vi "Flancos.vi"() -> ()   [LabVIEW 2017]
panel:
  out "Falling 4":dbl
  out "Rise 4":dbl
  out "Falling 3":dbl
  out "Rise 3":dbl
  out "Falling 2":dbl
  out "Rise 2":dbl
  out "Falling":dbl
  out "Rise":dbl
  in  "stop":bool
  in  "Alarma 4":bool
  in  "Alarma 3":bool
  in  "Alarma 2":bool
  in  "Alarma":bool
  out "Conteo 4":bool
  out "Conteo 3":bool
  out "Conteo 2":bool
  in  "stop 2":bool
  out "Waveform Chart":dbl(graph)
  in  "Seleccion":bool
  out "Conteo":bool
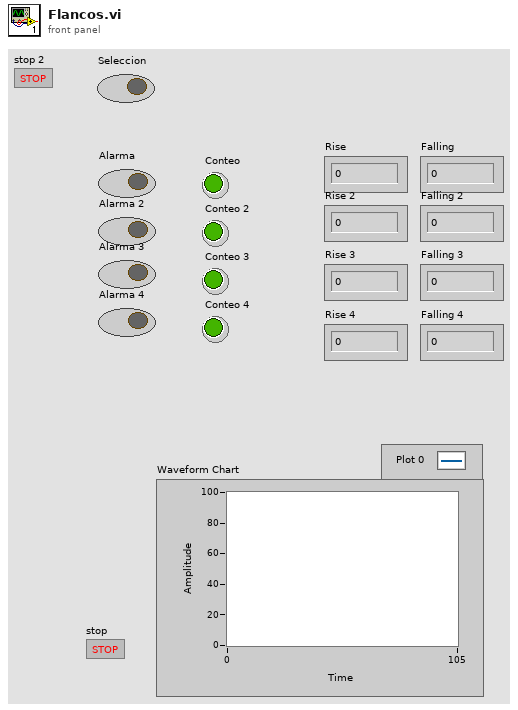
[diagram p1: front panel]
types:
  T1 = cluster{"Cont":i32, "Cont2":i32, "Cont3":i32, "Cont4":i32, "Bajada":i32, "Bajada 2":i32, "Bajada 3":i32, "Bajada 4":i32}
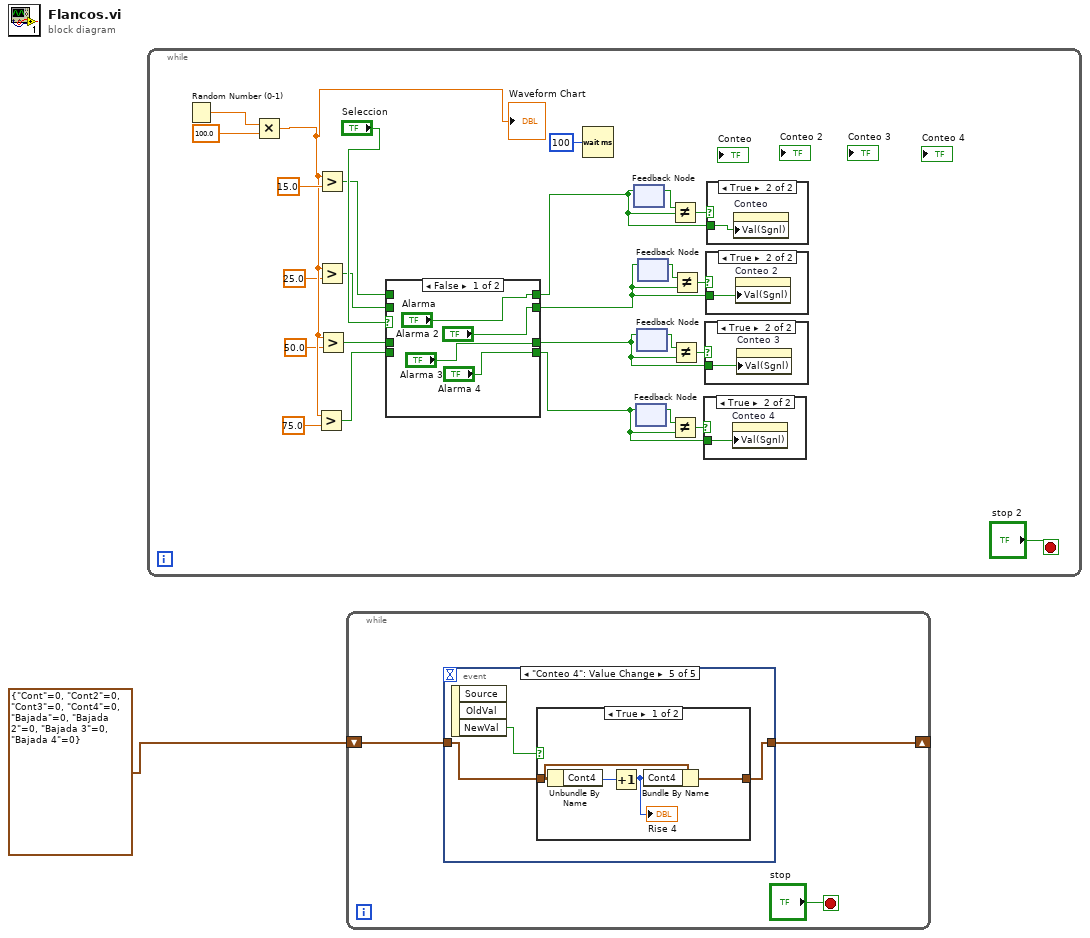
[diagram p0: block diagram]
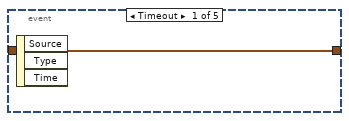
[diagram p2: hidden frame]
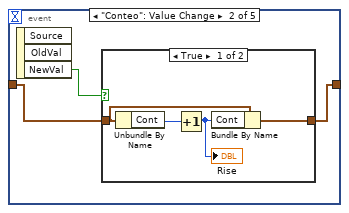
[diagram p3: hidden frame]
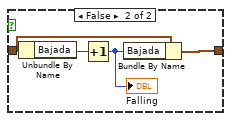
[diagram p4: hidden frame]
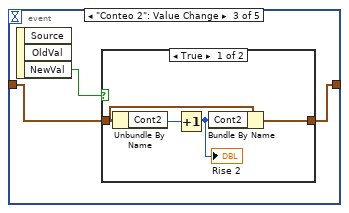
[diagram p5: hidden frame]
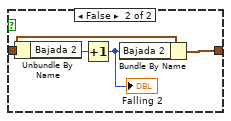
[diagram p6: hidden frame]
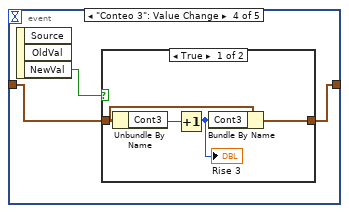
[diagram p7: hidden frame]
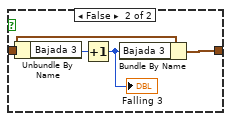
[diagram p8: hidden frame]
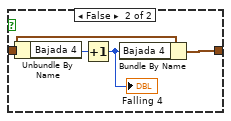
[diagram p9: hidden frame]
diagram:
  n1 = while {
    stop <- "stop 2" stop-if-true
    n2 = Random Number (0-1)() -> (number: 0 to 1=w27:dbl)
    n3 = Multiply(x=w27, y=100.0) -> (x*y=w20:dbl)
    "Waveform Chart" <- w20
    n4 = Greater?(x=w20, y=75.0) -> (0:w12:bool)
    n5 = Greater?(x=w20, y=15.0) -> (0:w15:bool)
    n6 = Greater?(x=w20, y=25.0) -> (0:w14:bool)
    n7 = Greater?(x=w20, y=50.0) -> (0:w13:bool)
    n8 = case shown="False" "Seleccion" {
      tunnel: w15 -> [_ w38]
      tunnel: w14 -> [_ w37]
      tunnel: w13 -> [_ w36]
      tunnel: w12 -> [_ w35]
      tunnel: ["Alarma" w38] -> w11
      tunnel: ["Alarma 2" w37] -> w8
      tunnel: ["Alarma 3" w36] -> w5
      tunnel: ["Alarma 4" w35] -> w2
      frame False {
      }
      frame True {
      }
    }
    n9 = Wait (ms)(milliseconds to wait=u32 100) -> ()  [unwired: 1 out]
    n10 = feedback-in #1(w11) -> ()
    n11 = feedback #1() -> (w22:bool)  [unwired: 1 in]
    n12 = feedback #2() -> (w4:bool)  [unwired: 1 in]
    n13 = feedback-in #2(w2) -> ()
    n14 = feedback #3() -> (w7:bool)  [unwired: 1 in]
    n15 = feedback-in #3(w5) -> ()
    n16 = feedback #4() -> (w10:bool)  [unwired: 1 in]
    n17 = feedback-in #4(w8) -> ()
    n18 = Not Equal?(x=w22, y=w11) -> (x != y?=w21:bool)
    n19 = Not Equal?(x=w4, y=w2) -> (x != y?=w3:bool)
    n20 = Not Equal?(x=w7, y=w5) -> (x != y?=w6:bool)
    n21 = Not Equal?(x=w10, y=w8) -> (x != y?=w9:bool)
    n22 = case shown="True" w3 {
      tunnel: w2 -> [_ w28]
      frame False {
      }
      frame True {
        n23 = property on="Conteo 4" class="Bool (strict)"("Val(Sgnl)"=w28) -> ()  [unwired: 2 in, 2 out]
      }
    }
    n24 = case shown="True" w6 {
      tunnel: w5 -> [_ w29]
      frame False {
      }
      frame True {
        n25 = property on="Conteo 3" class="Bool (strict)"("Val(Sgnl)"=w29) -> ()  [unwired: 2 in, 2 out]
      }
    }
    n26 = case shown="True" w9 {
      tunnel: w8 -> [_ w30]
      frame False {
      }
      frame True {
        n27 = property on="Conteo 2" class="Bool (strict)"("Val(Sgnl)"=w30) -> ()  [unwired: 2 in, 2 out]
      }
    }
    n28 = case shown="True" w21 {
      tunnel: w11 -> [_ w39]
      frame False {
      }
      frame True {
        n29 = property on="Conteo" class="Bool (strict)"("Val(Sgnl)"=w39) -> ()  [unwired: 2 in, 2 out]
      }
    }
  }
  n30 = while {
    shift-right: [w40] -> _
    shift-left: T1 {"Cont"=0, "Cont2"=0, "Cont3"=0, "Cont4"=0, "Bajada"=0, "Bajada 2"=0, "Bajada 3"=0, "Bajada 4"=0} -> [w42]
    stop <- "stop" stop-if-true
    n31 = event shown="[4] \"Conteo 4\": Value Change" {
      selector: _ -> [_ _ _ _ _]
      dyn-events: _ -> [_ _ _ _ _]
      timeout: _ -> [_ _ _ _ _]
      tunnel: w42 -> [w43 w46 w57 w68 w79]
      tunnel: [w43 w45 w56 w67 w78] -> w40
      event Timeout {
        n32 = event-data() -> ()  [unwired: 1 in, 3 out]
      }
      event "Conteo": Value Change {
        n33 = event-data() -> ("NewVal"=w44:bool)  [unwired: 1 in, 2 out]
        n34 = case shown="True" w44 {
          tunnel: w46 -> [w49 w53]
          tunnel: [w48 w52] -> w45
          frame True {
            n35 = Unbundle By Name(w49) -> ("Cont"=w50:i32)
            n36 = Increment(x=w50) -> (x+1=w47:i32)
            "Rise" <- w47
            n37 = Bundle By Name(cluster=w49, "Cont"=w47) -> (w48:T1)
          }
          frame False {
            n38 = Unbundle By Name(w53) -> ("Bajada"=w54:i32)
            n39 = Increment(x=w54) -> (x+1=w51:i32)
            "Falling" <- w51
            n40 = Bundle By Name(cluster=w53, "Bajada"=w51) -> (w52:T1)
          }
        }
      }
      event "Conteo 2": Value Change {
        n41 = event-data() -> ("NewVal"=w55:bool)  [unwired: 1 in, 2 out]
        n42 = case shown="True" w55 {
          tunnel: w57 -> [w60 w64]
          tunnel: [w59 w63] -> w56
          frame True {
            n43 = Unbundle By Name(w60) -> ("Cont2"=w61:i32)
            n44 = Increment(x=w61) -> (x+1=w58:i32)
            "Rise 2" <- w58
            n45 = Bundle By Name(cluster=w60, "Cont2"=w58) -> (w59:T1)
          }
          frame False {
            n46 = Unbundle By Name(w64) -> ("Bajada 2"=w65:i32)
            n47 = Increment(x=w65) -> (x+1=w62:i32)
            "Falling 2" <- w62
            n48 = Bundle By Name(cluster=w64, "Bajada 2"=w62) -> (w63:T1)
          }
        }
      }
      event "Conteo 3": Value Change {
        n49 = event-data() -> ("NewVal"=w66:bool)  [unwired: 1 in, 2 out]
        n50 = case shown="True" w66 {
          tunnel: w68 -> [w71 w75]
          tunnel: [w70 w74] -> w67
          frame True {
            n51 = Unbundle By Name(w71) -> ("Cont3"=w72:i32)
            n52 = Increment(x=w72) -> (x+1=w69:i32)
            "Rise 3" <- w69
            n53 = Bundle By Name(cluster=w71, "Cont3"=w69) -> (w70:T1)
          }
          frame False {
            n54 = Unbundle By Name(w75) -> ("Bajada 3"=w76:i32)
            n55 = Increment(x=w76) -> (x+1=w73:i32)
            "Falling 3" <- w73
            n56 = Bundle By Name(cluster=w75, "Bajada 3"=w73) -> (w74:T1)
          }
        }
      }
      event "Conteo 4": Value Change {
        n57 = event-data() -> ("NewVal"=w77:bool)  [unwired: 1 in, 2 out]
        n58 = case shown="True" w77 {
          tunnel: w79 -> [w82 w86]
          tunnel: [w81 w85] -> w78
          frame True {
            n59 = Unbundle By Name(w82) -> ("Cont4"=w83:i32)
            n60 = Increment(x=w83) -> (x+1=w80:i32)
            "Rise 4" <- w80
            n61 = Bundle By Name(cluster=w82, "Cont4"=w80) -> (w81:T1)
          }
          frame False {
            n62 = Unbundle By Name(w86) -> ("Bajada 4"=w87:i32)
            n63 = Increment(x=w87) -> (x+1=w84:i32)
            "Falling 4" <- w84
            n64 = Bundle By Name(cluster=w86, "Bajada 4"=w84) -> (w85:T1)
          }
        }
      }
    }
  }
